vi "_FPGA_AuxParamerConverter.vi"(9 "Parameter2 in":u64=1, 10 "Parameter1 in":u64=1) -> (0 "Cycle 2":u32=2147483648, 1 "Voltage2":fxp<+,14,14>, 2 "Cycle 1":u32=2147483648, 3 "Voltage1":fxp<+,14,14>, 5 "MaxCycle-1 out":u32=1)   [LabVIEW 2018]
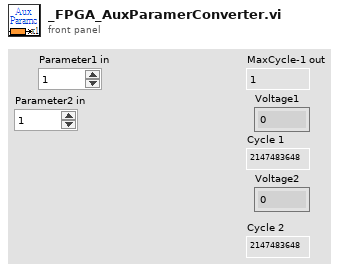
[diagram p1: front panel]
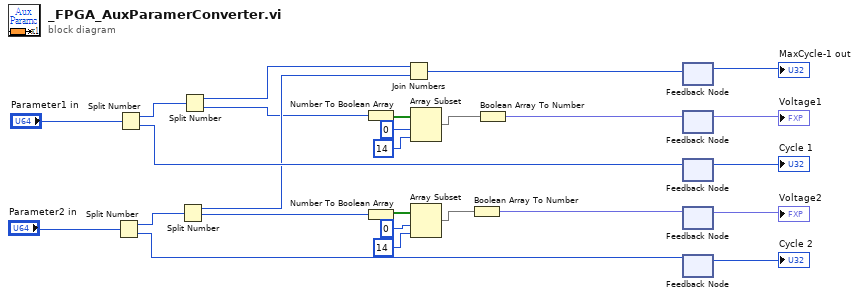
[diagram p0: block diagram]
diagram:
  n1 = Split Number(x="Parameter2 in") -> (hi(x)=w19:u32, lo(x)=w20:u32)
  n2 = Split Number(x="Parameter1 in") -> (hi(x)=w18:u32, lo(x)=w22:u32)
  n3 = Split Number(x=w19) -> (hi(x)=w16:u16, lo(x)=w7:u16)
  n4 = Split Number(x=w18) -> (hi(x)=w17:u16, lo(x)=w14:u16)
  n5 = Number To Boolean Array(number=w14) -> (Boolean array=w13:bool[])
  n6 = Number To Boolean Array(number=w7) -> (Boolean array=w8:bool[])
  n7 = Join Numbers(hi=w17, lo=w16) -> ((hi.lo)=w15:u32)
  n8 = Array Subset(array=w13, index=0, length=14) -> (w6:bool[])
  n9 = Array Subset(array=w8, index=0, length=14) -> (w3:bool[])
  n10 = Boolean Array To Number(Boolean array=w3) -> (number=w2:fxp<+,14,14>)
  n11 = Boolean Array To Number(Boolean array=w6) -> (number=w5:fxp<+,14,14>)
  n12 = feedback-in #1(w15) -> ()
  n13 = feedback #1() -> (→"MaxCycle-1 out":u32)  [unwired: 1 in]
  n14 = feedback #2() -> (→"Voltage1":fxp<+,14,14>)  [unwired: 1 in]
  n15 = feedback-in #2(w5) -> ()
  n16 = feedback #3() -> (→"Cycle 1":u32)  [unwired: 1 in]
  n17 = feedback-in #3(w22) -> ()
  n18 = feedback #4() -> (→"Voltage2":fxp<+,14,14>)  [unwired: 1 in]
  n19 = feedback-in #4(w2) -> ()
  n20 = feedback #5() -> (→"Cycle 2":u32)  [unwired: 1 in]
  n21 = feedback-in #5(w20) -> ()
